vi "PerfResize.vi"() -> ()   [LabVIEW 2024, in "POTTypedCircularBuffer.Tests.Perf.lvlib"]
uses:
  POTTypedCircularBuffer.Tests.Perf.lvlib
  POTTypedCircularBuffer.lvclass/POTTypedCircularBuffer.ctl
  <vilib>/Analysis/baseanly.llb/Mean (DBL).vi
  ReadCount.vi
  Reorder.vi
  <vilib>/Analysis/NI_AALBase.lvlib
  POTTypedCircularBuffer.lvclass
panel:
  out "resize time":dbl format="%.2p"
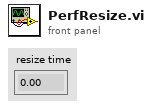
[diagram p1: front panel]
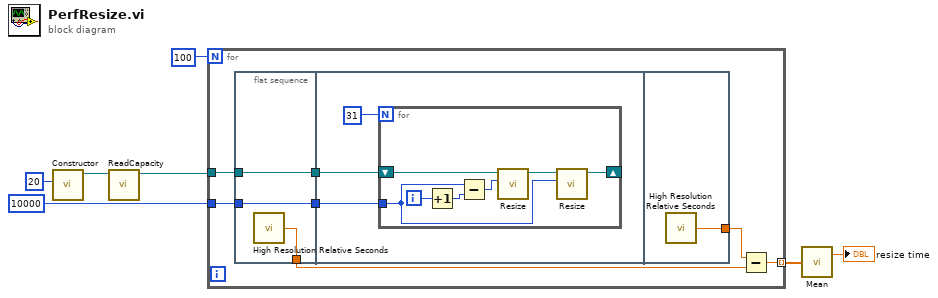
[diagram p0: block diagram]
diagram:
  n1 = call "Constructor.vi"("Capacity 2^n"=u32 20) -> ("POTTypedCircularBuffer out"=w3:refnum<class "POTTypedCircularBuffer.lvclass">)  [unwired: 10 in]
  n2 = call "ReadCapacity.vi"("POTTypedCircularBuffer in"=w3) -> ("POTTypedCircularBuffer out"=w2:refnum<class "POTTypedCircularBuffer.lvclass">)  [unwired: 9 in, 1 out]
  n3 = for {
    N: 100 -> [_]
    tunnel: w2 -> [w14]
    tunnel: [w10] -> w5 mode=indexing
    tunnel: u32 10000 ("Capacity") -> [w9]
    n4 = flat-sequence {
      tunnel: w14 -> [w17]
      tunnel: [w17] -> w13
      tunnel: [w16] -> w11
      tunnel: w9 -> [w15]
      tunnel: [w15] -> w8
      tunnel: w13 -> [w20]
      tunnel: w8 -> [w18]
      tunnel: [w28] -> w12
      frame #0 {
        n5 = call <vilib>:"High Resolution Relative Seconds.vi"() -> ("relative seconds"=w16:dbl)
      }
      frame #1 {
        n6 = for {
          N: 31 -> [_]
          shift-right: [w22] -> _
          shift-left: w20 -> [w25]
          tunnel: w18 -> [w23]
          i -> [w27]
          n7 = Increment(x=w27) -> (x+1=w26:i32)
          n8 = Subtract(x=w23, y=w26) -> (x-y=w21:u32)
          n9 = call "Resize.vi"("Capacity 2^n"=w21, "POTTypedCircularBuffer in"=w25) -> ("POTTypedCircularBuffer out"=w24:refnum<class "POTTypedCircularBuffer.lvclass">)  [unwired: 9 in]
          n10 = call "Resize.vi"("Capacity 2^n"=w23, "POTTypedCircularBuffer in"=w24) -> ("POTTypedCircularBuffer out"=w22:refnum<class "POTTypedCircularBuffer.lvclass">)  [unwired: 9 in]
        }
      }
      frame #2 {
        n11 = call <vilib>:"High Resolution Relative Seconds.vi"() -> ("relative seconds"=w28:dbl)
      }
    }
    n12 = Subtract(x=w12, y=w11) -> (x-y=w10:dbl)
  }
  n13 = call-poly <vilib>:"Mean.vi"("X"=w5) -> ("mean"=→"resize time":dbl)  [unwired: 1 out]
